vi "SR830_highfreq_readout_2.vi"(0 "address string":string="30", 1 "X channel":tag="Dev2/ai0", 5 "number of samples per channel":i32=50000, 7 "sample mode":i32(ring)=10178 items=["Finite Samples"=10178, "Continuous Samples"=10123], 9 "rate":dbl=5000.0 format="%0.2f", 11 "error in (no error)":errorcluster, 12 "Y channel":tag="Dev2/ai1", 13 "Dc Voltage (V)":dbl=1.0 format="%0.2f") -> (2 "Lock In Signal Spectrum (mV/V) X,Y,R":cluster{"f0":dbl, "df":dbl, "magnitude":dbl[]}[](graph), 3 "Lockin R (mV/V)":waveform(dbl)(graph), 4 "Lock In Signal Spectrum (mV/V)":cluster{"f0":dbl, "df":dbl, "magnitude":dbl[]}(graph), 6 "Lock_in R (mV/V)":dbl[](graph), 8 "Lockin X,Y,R (mV/V)":waveform(dbl)[](graph), 10 "Theta":dbl[](graph), 14 "Lockin Theta":waveform(dbl)(graph), 15 "error out":errorcluster)   [LabVIEW 2013]
uses:
  <vilib>/DAQmx/read.llb/DAQmx Read (Analog 1D DBL 1Chan NSamp).vi
  <vilib>/DAQmx/read.llb/DAQmx Read (Analog 2D DBL NChan NSamp).vi
  <vilib>/DAQmx/create/channels.llb/DAQmx Create Channel (AI-Voltage-Basic).vi
  <vilib>/DAQmx/configure/timing.llb/DAQmx Timing (Sample Clock).vi
  <vilib>/DAQmx/miscellaneous.llb/DAQmx Fill In Error Info.vi
  <vilib>/express/express analysis/Spectral/Block/exnSpectralBlock spectral measurements peak poly.vi
  <vilib>/express/express analysis/Spectral/Block/exnSpectralBlock spectral measurements peak array WFM.vi
  <vilib>/express/express analysis/Spectral/Block/exnSpectralBlock spectral measurements peak WFM.vi
  <vilib>/express/express analysis/Spectral/XNode/ExpressSpectralMeasurementsBlockNode.xnode
  <resource>/objmgr/daqmx.rc
panel:
  in  "Ref channels":tag="Dev1/ai3"
  out "Y":dbl[](array[numeric])
  out "X":dbl[](array[numeric])
  in  "minimum value":dbl=-10.0 format="%0.2f"
  in  "maximum value":dbl=10.0 format="%0.2f"
  in  "stop":bool
  out "Sensitivity":dbl
  in  "Tab Control":enum32{"Page 1", "Spectrum", "Page 2"}(tab)
  out "Ref  2f":waveform(dbl)(graph)
  out "Ref":dbl[](graph)
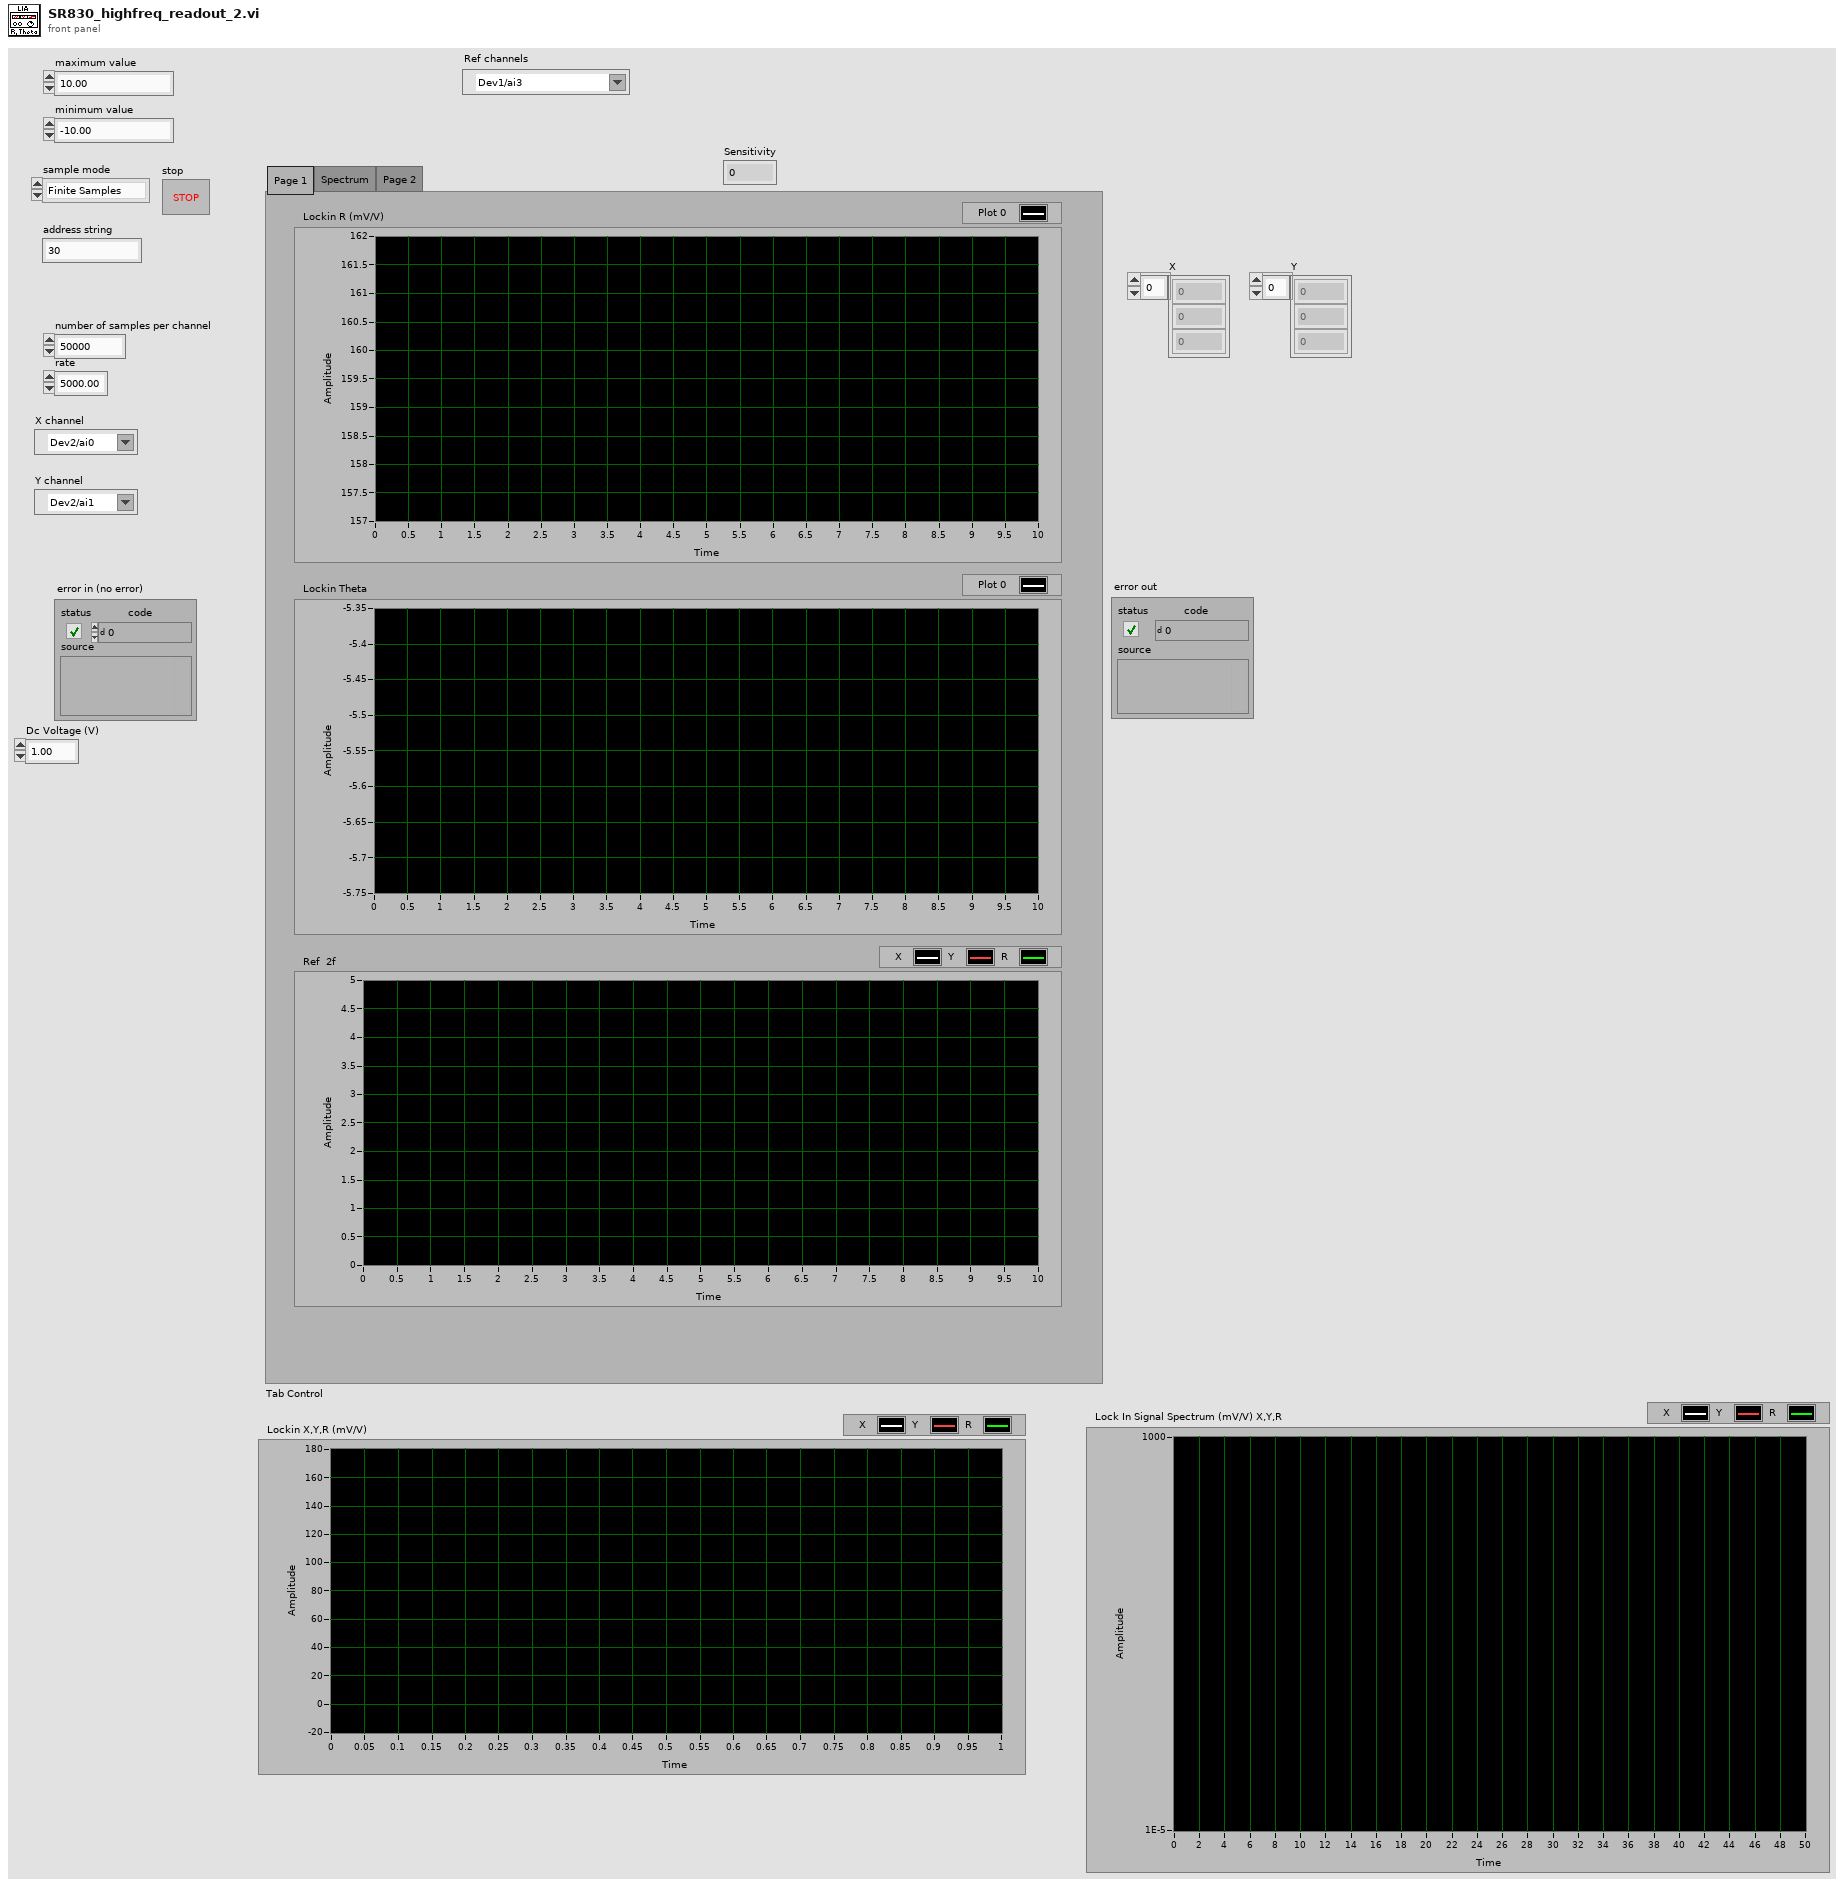
[diagram p1: front panel]
types:
  T1 = cluster{"averaging mode":u16, "weighting mode":u16, "number of averages":u32}
  T2 = cluster{"dB On (F)":bool, "unwrap phase (F)":bool, "convert to degree (F)":bool}
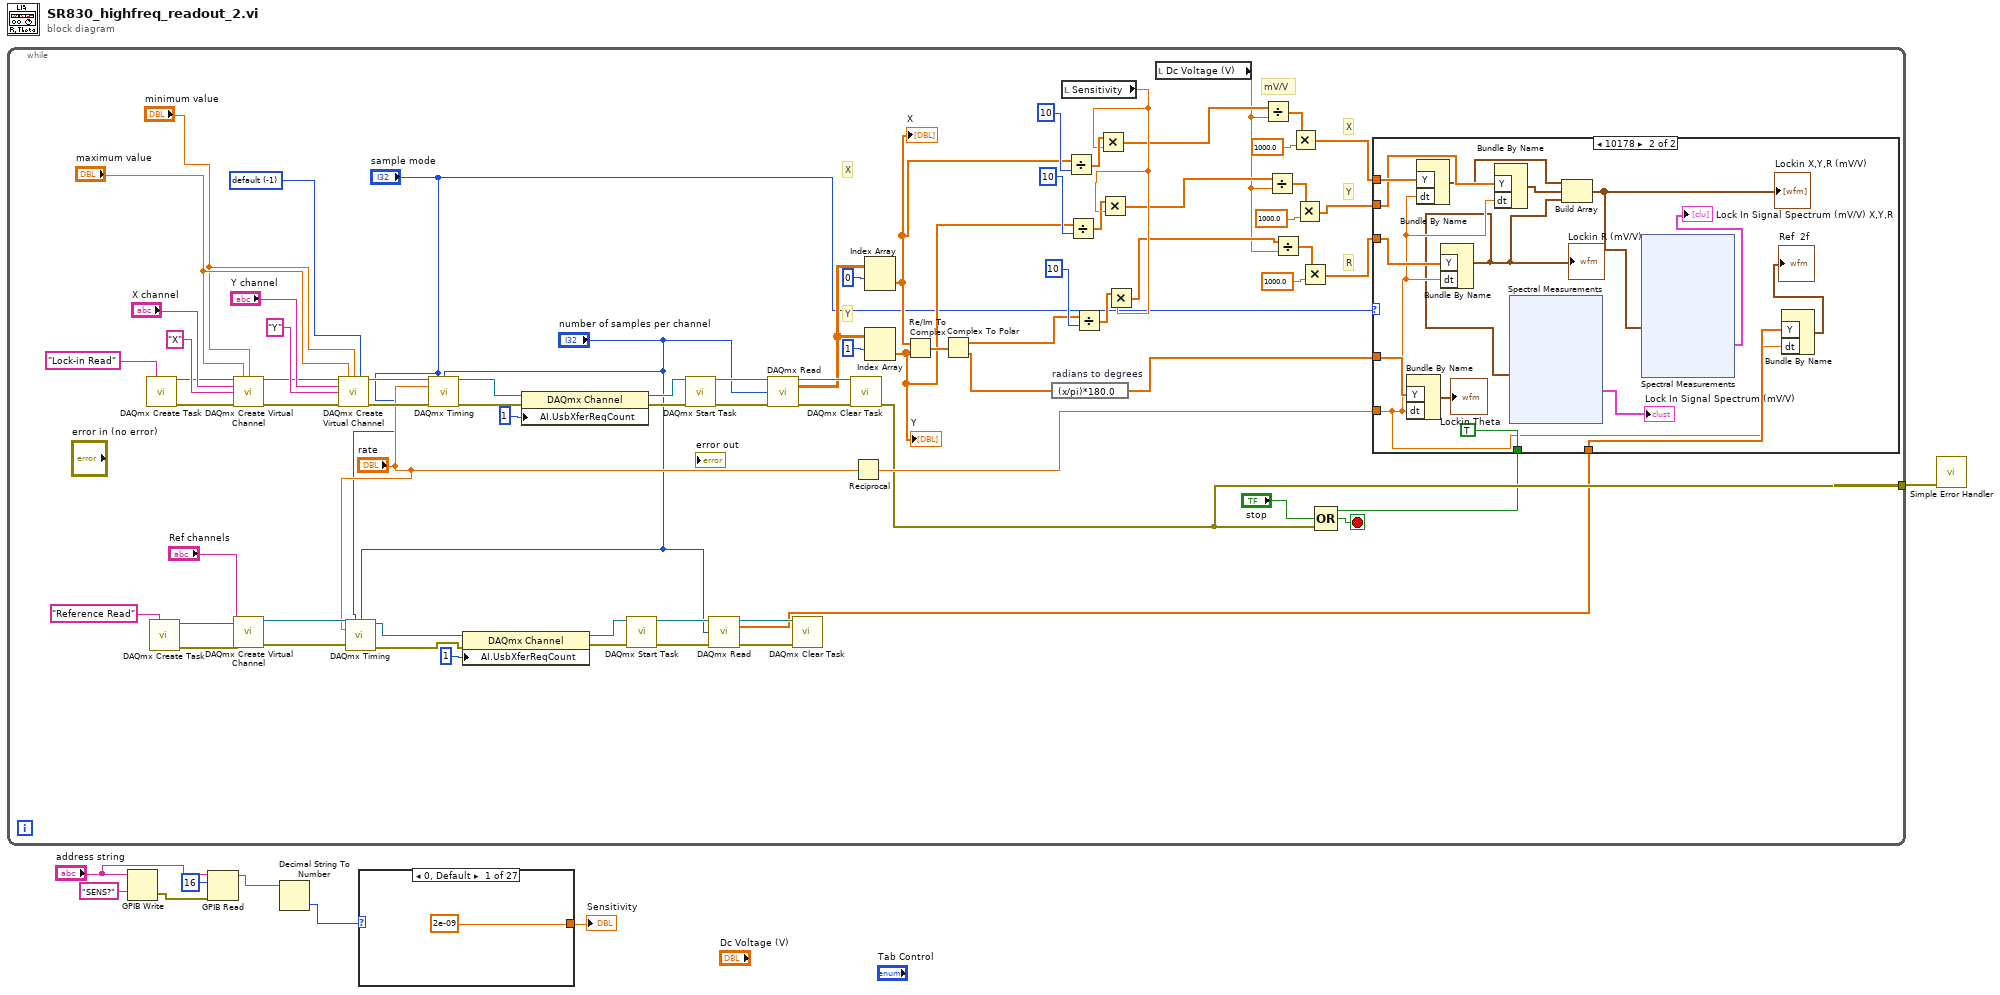
[diagram p0: block diagram]
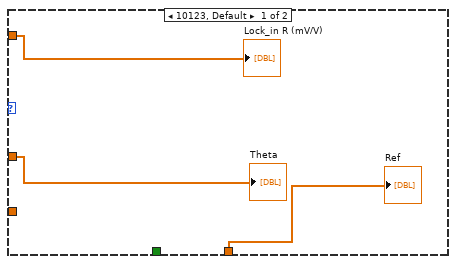
[diagram p2: hidden frame]
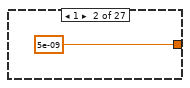
[diagram p3: hidden frame]
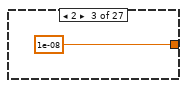
[diagram p4: hidden frame]
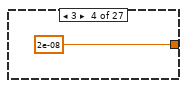
[diagram p5: hidden frame]
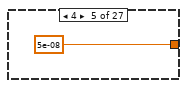
[diagram p6: hidden frame]
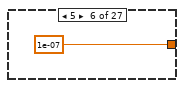
[diagram p7: hidden frame]
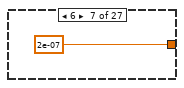
[diagram p8: hidden frame]
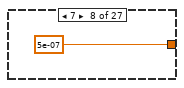
[diagram p9: hidden frame]
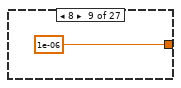
[diagram p10: hidden frame]
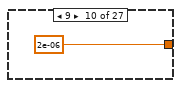
[diagram p11: hidden frame]
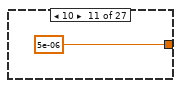
[diagram p12: hidden frame]
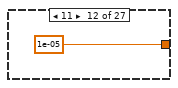
[diagram p13: hidden frame]
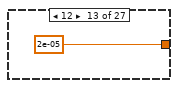
[diagram p14: hidden frame]
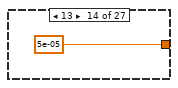
[diagram p15: hidden frame]
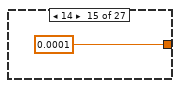
[diagram p16: hidden frame]
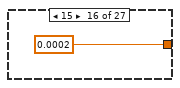
[diagram p17: hidden frame]
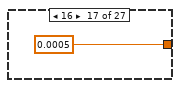
[diagram p18: hidden frame]
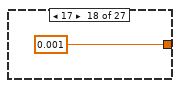
[diagram p19: hidden frame]
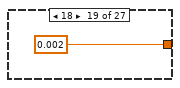
[diagram p20: hidden frame]
diagram:
  n1 = while {
    tunnel: [w52] -> w1
    stop <- w53 stop-if-true
    w67 = -1 items=["default"=-1, "RSE"=10083, "NRSE"=10078, "Differential"=10106, "Pseudodifferential"=12529] ("input terminal configuration")
    # "mV/V"
    # "R"
    # "Y"
    # "X"
    # "Y"
    # "X"
    n2 = call <vilib>:"DAQmx Create Task.vi"("new task name"="Lock-in Read") -> ("task out"=w74:refnum<k21>, "error out"=w73:errorcluster)  [unwired: 13 in]
    n3 = call <vilib>:"DAQmx Create Task.vi"("new task name"="Reference Read") -> ("task out"=w19:refnum<k21>, "error out"=w16:errorcluster)  [unwired: 13 in]
    n4 = call-poly <vilib>:"DAQmx Create Virtual Channel.vi"("task in"=w74, "maximum value"="maximum value", "minimum value"="minimum value", "physical channels"="X channel", "name to assign"="X", "error in"=w73) -> ("task out"=w75:refnum<k21>, "error out"=w76:errorcluster)  [unwired: 8 in]
    n5 = call-poly <vilib>:"DAQmx Create Virtual Channel.vi"("task in"=w19, "physical channels"="Ref channels", "error in"=w16) -> ("task out"=w18:refnum<k21>, "error out"=w15:errorcluster)  [unwired: 11 in]
    n6 = call-poly <vilib>:"DAQmx Create Virtual Channel.vi"("task in"=w75, "maximum value"="maximum value", "minimum value"="minimum value", "input terminal configuration"=w67, "physical channels"="Y channel", "name to assign"="Y", "error in"=w76) -> ("task out"=w83:refnum<k21>, "error out"=w84:errorcluster)  [unwired: 7 in]
    n7 = call-poly <vilib>:"DAQmx Timing.vi"("task/channels in"=w18, "sample mode"="sample mode", "samples per channel"="number of samples per channel", "rate"="rate", "error in"=w15) -> ("task out"=w20:refnum<k21>, "error out"=w14:errorcluster)  [unwired: 9 in]
    n8 = call-poly <vilib>:"DAQmx Timing.vi"("task/channels in"=w83, "sample mode"="sample mode", "samples per channel"="number of samples per channel", "rate"="rate", "error in"=w84) -> ("task out"=w69:refnum<k21>, "error out"=w71:errorcluster)  [unwired: 9 in]
    n9 = property class="DAQmx Channel"(reference=w20, error in=w14, "AI.UsbXferReqCount"=u32 1) -> (reference out=w25:refnum<k21>, error out=w24:errorcluster)
    n10 = property class="DAQmx Channel"(reference=w69, error in=w71, "AI.UsbXferReqCount"=u32 1) -> (reference out=w68:refnum<k21>, error out=w70:errorcluster)
    n11 = call <vilib>:"DAQmx Start Task.vi"("task/channels in"=w25, "error in"=w24) -> ("task out"=w22:refnum<k21>, "error out"=w21:errorcluster)  [unwired: 12 in]
    n12 = call <vilib>:"DAQmx Start Task.vi"("task/channels in"=w68, "error in"=w70) -> ("task out"=w81:refnum<k21>, "error out"=w82:errorcluster)  [unwired: 12 in]
    n13 = call-poly <vilib>:"DAQmx Read.vi"("task/channels in"=w22, "number of samples per channel"="number of samples per channel", "error in"=w21) -> ("task out"=w27:refnum<k21>, "data"=w9:dbl[], "error out"=w26:errorcluster)  [unwired: 10 in]
    n14 = call-poly <vilib>:"DAQmx Read.vi"("task/channels in"=w81, "number of samples per channel"="number of samples per channel", "error in"=w82) -> ("task out"=w64:refnum<k21>, "data"=w62:dbl[][], "error out"=w65:errorcluster)  [unwired: 10 in]
    n15 = call <vilib>:"DAQmx Clear Task.vi"("task in"=w27, "error in"=w26) -> ()  [unwired: 13 in, 1 out]
    n16 = call <vilib>:"DAQmx Clear Task.vi"("task in"=w64, "error in"=w65) -> ("error out"=w52:errorcluster)  [unwired: 13 in]
    n17 = Reciprocal(x="rate") -> (1/x=w59:dbl)
    n18 = Index Array(array=w62, index (row)=0) -> (element=w43:dbl[])  [unwired: 1 in]
    "X" <- w43
    n19 = Index Array(array=w62, index (row)=1) -> (element=w42:dbl[])  [unwired: 1 in]
    "Y" <- w42
    n20 = Re/Im To Complex(1:w42, 2:w43) -> (0:w60:cdb[])
    n21 = Complex To Polar(r * e^(i*theta)=w60) -> (r=w48:dbl[], theta=w58:dbl[])
    n22 = expression code="(x/pi)*180.0" "radians to degrees"(w58) -> (w57:dbl[])
    n23 = local read "Sensitivity"() -> (w41:dbl)
    n24 = Divide(x=w43, y=10 ("Waveform")) -> (x/y=w44:dbl[])
    n25 = Divide(x=w42, y=10 ("Waveform")) -> (x/y=w47:dbl[])
    n26 = Divide(x=w48, y=10 ("Waveform")) -> (x/y=w55:dbl[])
    n27 = Multiply(x=w44, y=w41) -> (x*y=w39:dbl[])
    n28 = Multiply(x=w47, y=w41) -> (x*y=w34:dbl[])
    n29 = Multiply(x=w55, y=w41) -> (x*y=w30:dbl[])
    n30 = local read "Dc Voltage (V)"() -> (w28:dbl)
    n31 = Divide(x=w39, y=w28) -> (x/y=w38:dbl[])
    n32 = Divide(x=w34, y=w28) -> (x/y=w36:dbl[])
    n33 = Divide(x=w30, y=w28) -> (x/y=w31:dbl[])
    n34 = Multiply(x=w38, y=1000.0 ("rate")) -> (x*y=w37:dbl[])
    n35 = Multiply(x=w36, y=1000.0 ("rate")) -> (x*y=w33:dbl[])
    n36 = Multiply(x=w31, y=1000.0 ("rate")) -> (x*y=w29:dbl[])
    n37 = case shown="10178" "sample mode" {
      tunnel: w59 -> [_ w91]
      tunnel: w57 -> [w87 w99]
      tunnel: w29 -> [w86 w98]
      tunnel: [_ TRUE ("value")] -> w49
      tunnel: w37 -> [_ w97]
      tunnel: w33 -> [_ w96]
      tunnel: w9 -> [w85 w92]
      frame 10123, Default {
        "Lock_in R (mV/V)" <- w86
        "Theta" <- w87
        "Ref" <- w85
      }
      frame 10178 {
        n38 = Bundle By Name("Y"=w99, "dt"=w91) -> (→"Lockin Theta":waveform(dbl))  [unwired: 1 in]
        n39 = Bundle By Name("Y"=w97, "dt"=w91) -> (w95:waveform(dbl))  [unwired: 1 in]
        n40 = Bundle By Name("Y"=w98, "dt"=w91) -> (w89:waveform(dbl))  [unwired: 1 in]
        "Lockin R (mV/V)" <- w89
        n41 = Bundle By Name("Y"=w96, "dt"=w91) -> (w90:waveform(dbl))  [unwired: 1 in]
        n42 = xnode "Spectral Measurements"("Signals"=w89) -> ("FFT - (Peak)"=→"Lock In Signal Spectrum (mV/V)":cluster{"f0":dbl, "df":dbl, "magnitude":dbl[]})  [unwired: 1 in, 2 out]
        n43 = Build Array(w95, w90, w89) -> (w94:waveform(dbl)[])
        "Lockin X,Y,R (mV/V)" <- w94
        n44 = xnode "Spectral Measurements"("Signals"=w94) -> ("FFT - (Peak)"=→"Lock In Signal Spectrum (mV/V) X,Y,R":cluster{"f0":dbl, "df":dbl, "magnitude":dbl[]}[])  [unwired: 1 in, 2 out]
        n45 = Bundle By Name("Y"=w92, "dt"=w91) -> (→"Ref  2f":waveform(dbl))  [unwired: 1 in]
      }
    }
    n46 = Compound Arithmetic op=OR(w49, "stop", w52) -> (w53:bool)
  }
  n47 = GPIB Write(0:"address string", 1:"SENS?" ("data")) -> (6:w7:errorcluster)  [unwired: 3 in, 1 out]
  n48 = GPIB Read(0:"address string", 1:16 ("byte count"), 3:w7) -> (5:w5:string)  [unwired: 2 in, 2 out]
  n49 = Decimal String To Number(string=w5) -> (number=w3:i32)  [unwired: 2 in, 1 out]
  n50 = case shown="0, Default" w3 {
    tunnel: [2e-09 5e-09 1e-08 2e-08 5e-08 1e-07 2e-07 5e-07 1e-06 2e-06 5e-06 1e-05 2e-05 5e-05 0.0001 0.0002 0.0005 0.001 0.002 0.005 0.01 0.02 0.05 0.1 0.2 0.5 1] -> w2
    frame 0, Default {
    }
    frame 1 {
    }
    frame 2 {
    }
    frame 3 {
    }
    frame 4 {
    }
    frame 5 {
    }
    frame 6 {
    }
    frame 7 {
    }
    frame 8 {
    }
    frame 9 {
    }
    frame 10 {
    }
    frame 11 {
    }
    frame 12 {
    }
    frame 13 {
    }
    frame 14 {
    }
    frame 15 {
    }
    frame 16 {
    }
    frame 17 {
    }
    frame 18 {
    }
    frame 19 {
    }
    frame 20 {
    }
    frame 21 {
    }
    frame 22 {
    }
    frame 23 {
    }
    frame 24 {
    }
    frame 25 {
    }
    frame 26 {
    }
  }
  "Sensitivity" <- w2
  n51 = call <vilib>:"Simple Error Handler.vi"("error in (no error)"=w1) -> ()  [unwired: 4 in, 5 out]
